vi "Actor Core.vi"(8 "error in":errorcluster, 11 "Hardware Buzzer in":refnum<class "Simulated Hardware.lvclass">) -> (0 "error out":errorcluster, 3 "Actor out":refnum<class "Actor.lvclass">)   [LabVIEW 2024, in "Simulated Hardware.lvlib" / "Simulated Hardware.lvclass"]
doc: "<p>(<strong>Filename</strong>: <span class=\"dnl\">Actor Framework.lvlib:Actor.lvclass:Actor Core.vi</span>)</p>\n<p>Receives messages to the actor, reacts to them, and initiates any error handling that may shut the actor down.</p>\n<p>Descendant classes may override this VI to append parallel tasks for the actor to complete while it handles messages. Overrides use the <a href=\"nihelplauncher://docs/csh?context=lvcore_glang_udclass\">Call Parent Class Method</a> node.</p>"
uses:
  Simulated Hardware.lvclass
  Simulated Hardware.lvclass/Simulated Hardware.ctl
  <vilib>/ActorFramework/Actor/Actor.lvclass
  <vilib>/ActorFramework/Stop Msg/Stop Msg.lvclass
  C:/Program Files/National Instruments/LabVIEW 2024/vi.lib/ActorFramework/Actor/Actor.lvclass
  Controller/Controller Messages/Buzzer Pressed Msg/Buzzer Pressed Msg.lvclass
  Controller/Controller Messages/Set DAQ Panel Reference Msg/Set DAQ Panel Reference Msg.lvclass
panel:
  in  "Stop":bool
  in  "3":bool
  in  "2":bool
  in  "1":bool
  in  "0":bool
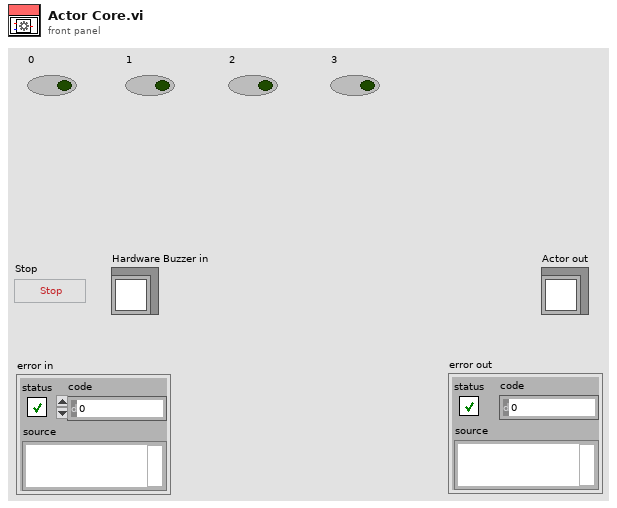
[diagram p1: front panel]
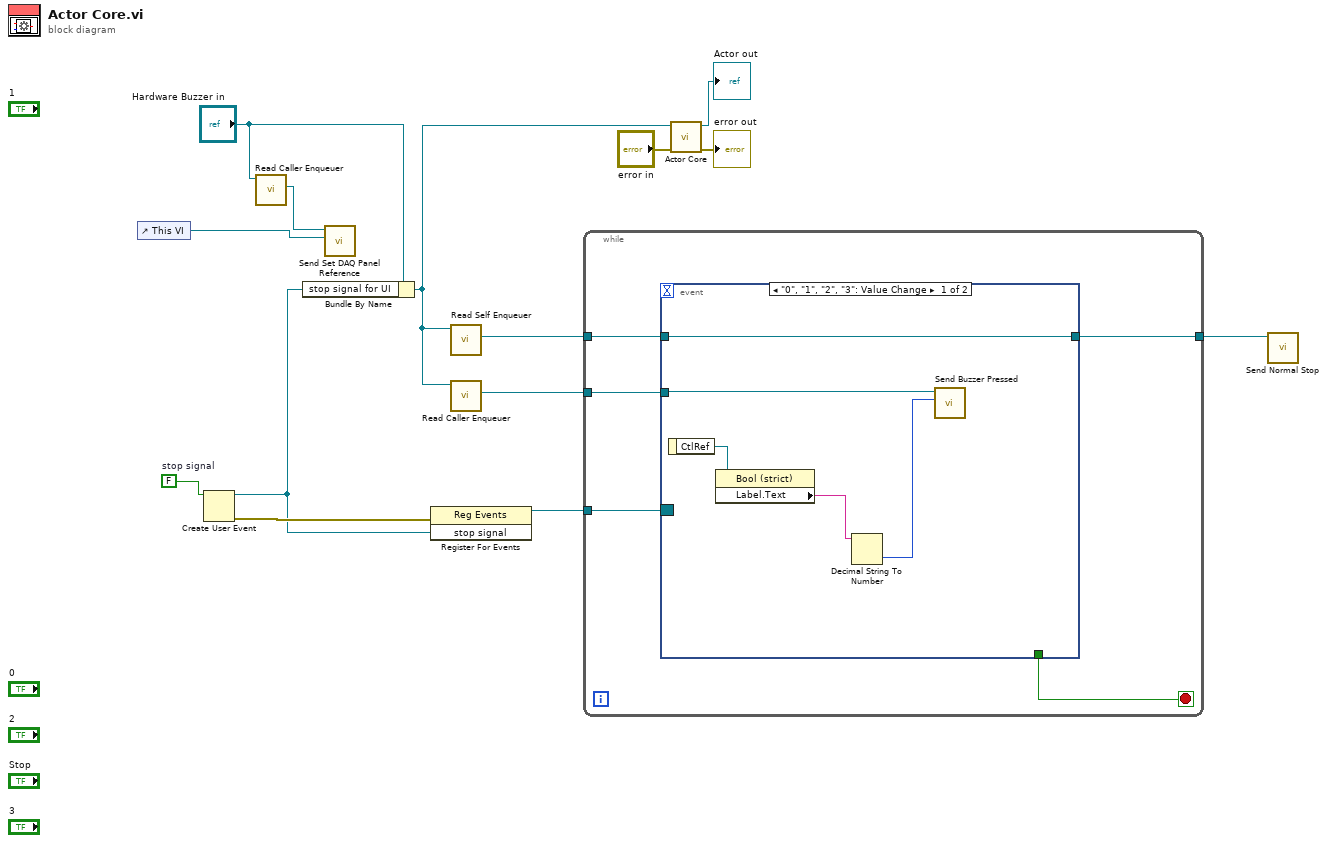
[diagram p0: block diagram]
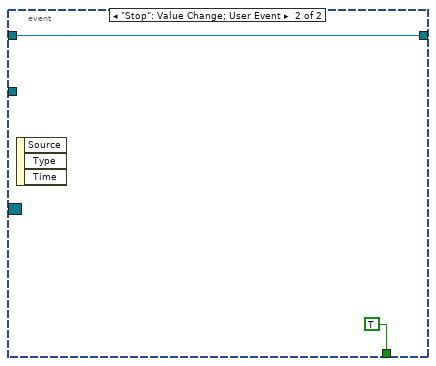
[diagram p2: hidden frame]
diagram:
  w7 = FALSE  # stop signal
  n1 = control-ref of="This VI"() -> (w1:refnum<vi>)
  n2 = Create User Event(user event datatype=w7) -> (user event=w8:refnum<user-event>, error out=w9:errorcluster)  [unwired: 1 in]
  n3 = call <vilib>:"Read Caller Enqueuer.vi"("Actor"="Hardware Buzzer in") -> ("Caller Enqueuer"=w2:refnum<class "Message Enqueuer.lvclass">)  [unwired: 10 in]
  n4 = Bundle By Name(cluster="Hardware Buzzer in", "stop signal for UI"=w8) -> (w5:refnum<class "Simulated Hardware.lvclass">)
  n5 = call "Send Set DAQ Panel Reference.vi"("DAQ VI Reference"=w1, "Message Enqueuer"=w2) -> ()  [unwired: 8 in, 2 out]
  n6 = register-events(error in=w9, w8) -> (reference out=w6:refnum<event-registration>)  [unwired: 1 in, 1 out]
  n7 = call <vilib>:"Read Self Enqueuer.vi"("Actor"=w5) -> ("Self Enqueuer"=w11:refnum<class "Message Enqueuer.lvclass">)  [unwired: 10 in]
  n8 = call <vilib>:"Read Caller Enqueuer.vi"("Actor"=w5) -> ("Caller Enqueuer"=w4:refnum<class "Message Enqueuer.lvclass">)  [unwired: 10 in]
  n9 = while {
    tunnel: w11 -> [w18]
    tunnel: [w17] -> w10
    tunnel: w6 -> [w16]
    tunnel: w4 -> [w15]
    stop <- w19 stop-if-true
    n10 = event shown="[0] \"0\", \"1\", \"2\", \"3\": Value Change" {
      selector: w16 -> [_ _]
      dyn-events: _ -> [_ _]
      timeout: _ -> [_ _]
      tunnel: [_ TRUE] -> w19
      tunnel: w18 -> [w22 w25]
      tunnel: [w22 w25] -> w17
      tunnel: w15 -> [w21 _]
      event "0", "1", "2", "3": Value Change {
        n11 = event-data() -> ("CtlRef"=w24:refnum<vi>)  [unwired: 1 in]
        n12 = property class="Bool (strict)"(reference=w24) -> ("Label.Text"=w23:string)  [unwired: 1 in, 2 out]
        n13 = Decimal String To Number(string=w23) -> (number=w20:i32)  [unwired: 2 in, 1 out]
        n14 = call "Send Buzzer Pressed.vi"("Buzzer"=w20, "Message Enqueuer"=w21) -> ()  [unwired: 8 in, 2 out]
      }
      event "Stop": Value Change; User Event {
        n15 = event-data() -> ()  [unwired: 1 in, 3 out]
      }
    }
  }
  n16 = call-parent "Actor Core.vi"("error in"="error in", "Actor in"=w5) -> ("error out"=→"error out":errorcluster, "Actor out"=→"Actor out":refnum<class "Actor.lvclass">)  [unwired: 8 in]
  n17 = call <vilib>:"Send Normal Stop.vi"("Message Enqueuer"=w10) -> ()  [unwired: 10 in, 1 out]
